vi "Defer Front Panel.vi"(8 "error in (no error)":errorcluster, 11 "Message Maker in":refnum<class "Message Maker.lvclass">) -> (0 "error out":errorcluster, 3 "Message Maker out":refnum<class "Message Maker.lvclass">)   [LabVIEW 2023, in "Message Maker.lvclass"]
doc: "Toggles the defer panel updates for the main UI\n\nAuthor: Derek Trepanier\nCopyright: MGI 2015"
uses:
  Message Maker.lvclass
  Message Maker.lvclass/Message Maker.ctl
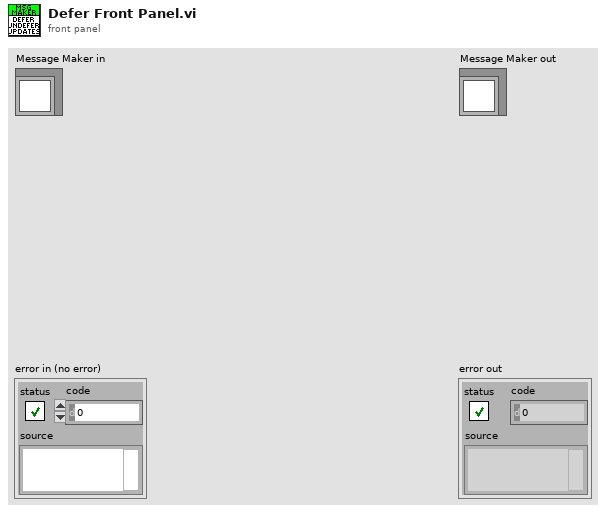
[diagram p1: front panel]
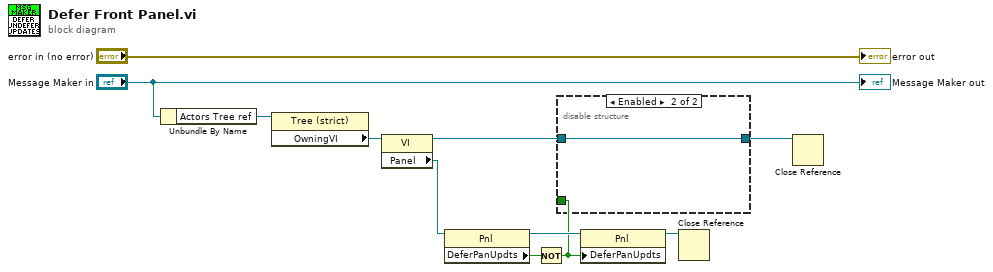
[diagram p0: block diagram]
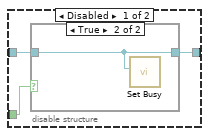
[diagram p2: hidden frame]
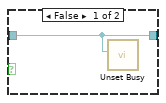
[diagram p3: hidden frame]
diagram:
  n1 = Unbundle By Name("Message Maker in") -> ("Actors Tree ref"=w8:refnum<vi>)
  n2 = property class="Tree (strict)"(reference=w8) -> ("OwningVI"=w9:refnum<vi>)  [unwired: 1 in, 2 out]
  n3 = property class="VI"(reference=w9) -> (reference out=w3:refnum<vi>, "Panel"=w7:refnum<vi>)  [unwired: 1 in, 1 out]
  n4 = property class="Pnl"(reference=w7) -> (reference out=w6:refnum<vi>, "DeferPanUpdts"=w5:bool)  [unwired: 1 in, 1 out]
  n5 = Not(x=w5) -> (.not. x?=w2:bool)
  n6 = disable-structure shown="Enabled" {
    disable-tunnel: w3 -> [w14 w17]
    disable-tunnel: w2 -> [w13 _]
    disable-tunnel: [w12 w17] -> w1
    frame Disabled {
      n7 = case shown="True" w13 {
        tunnel: w14 -> [w15 w16]
        tunnel: [w15 w16] -> w12
        frame False {
          n8 = call <vilib>:"Unset Busy.vi"("VI reference (current VI)"=w15) -> ()  [unwired: 10 in, 1 out]
        }
        frame True {
          n9 = call <vilib>:"Set Busy.vi"("VI reference (current VI)"=w16) -> ()  [unwired: 9 in, 2 out]
        }
      }
    }
    frame Enabled {
    }
  }
  n10 = property class="Pnl"(reference=w6, "DeferPanUpdts"=w2) -> (reference out=w4:refnum<vi>)  [unwired: 1 in, 1 out]
  n11 = Close Reference(reference=w4) -> ()  [unwired: 1 in, 1 out]
  n12 = Close Reference(reference=w1) -> ()  [unwired: 1 in, 1 out]
  "error out" <- "error in (no error)"
  "Message Maker out" <- "Message Maker in"
